vi "Swerve Drive t.vi"() -> ()   [LabVIEW 2017]
uses:
  Public/Documents/Cross The Road Electronics/Phoenix-LabVIEW/Motor Controller/Controls/CTRE_Phoenix_MotorControl_ControlMode.ctl
  <vilib>/Rock Robotics/WPI/ThirdParty/Phoenix-LabVIEW/Pigeon IMU/CTRE_PigeonIMU_TareType.ctl
  <extravilib>/ChannelInstances/Tag-dbl/Read With Abort.vi
  <extravilib>/ChannelInstances/Tag-a[.](dbl)/Read With Abort.vi
  <extravilib>/ChannelInstances/Tag-a[.](dbl)/Write With Abort.vi
  <extravilib>/ChannelInstances/Tag-dbl/Write With Abort.vi
  <extravilib>/ChannelInstances/Tag-dbl/Instantiate.vi
  <vilib>/Rock Robotics/Network Tables/NT Read Number.vi
  Robot Global Data.vi
  <extravilib>/ChannelInstances/Tag-dbl/Endpoint.vi
  <vilib>/Rock Robotics/WPI/ThirdParty/Phoenix-LabVIEW/Pigeon IMU/CTRE_PigeonIMU_GetYPR.vi
  <vilib>/Rock Robotics/Network Tables/NT Write Number.vi
  <extravilib>/ChannelInstances/Tag-a[.](dbl)/Instantiate.vi
  <extravilib>/ChannelInstances/Tag-dbl/EndpointRead.vi
  <vilib>/Rock Robotics/WPI/ThirdParty/Phoenix-LabVIEW/Motor Controller/Get/CTRE_Phoenix_MotorController_GetSelectedSensorData.vi
  <extravilib>/ChannelInstances/Tag-a[.](dbl)/Endpoint.vi
  <vilib>/Rock Robotics/Network Tables/NT Write Numeric Array.vi
  <extravilib>/ChannelInstances/Tag-a[.](dbl)/EndpointRead.vi
  <vilib>/addons/control/pid/pid.llb/PID (DBL).vi
  <extravilib>/ChannelInstances/Tag-dbl.lvlib
  <extravilib>/ChannelInstances/Tag-a[.](dbl).lvlib
  <vilib>/ptbypt/NI_PtbyPt.lvlib
  <vilib>/addons/control/pid/NI_PID_pid.lvlib
panel:
  in  "Limelight PID gains":T1={"proportional gain (Kc)"=0.035, "integral time (Ti, min)"=0.0, "derivative time (Td, min)"=0.0}
  out "Loop 3":u32=30
  out "Loop 2":u32=30
  out "Loop 1":u32=20
  in  "Rot. Point X":dbl
  in  "Rot. Point Y":dbl
  in  "Robot Width":dbl=21.125
  in  "Robot Length":dbl=22.0
  # "SWERVE DRIVE\nVersion 6.2\nCory Lynch\nChris Garuti\nGavin Popkin\nKaitlyn Sandor\nApple Pi Robotics\nTeam 2067"
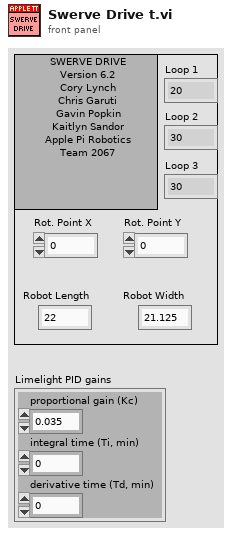
[diagram p1: front panel]
types:
  T1 = cluster{"proportional gain (Kc)":dbl, "integral time (Ti, min)":dbl, "derivative time (Td, min)":dbl}
  T2 = typedef "CTRE_PigeonIMU_DeviceRef.ctl" = cluster{"DeviceStatus":errorcluster, "Device Number":u8, "Type":T3, "Device ID":u32, "Handle":u64, "UsageFrame":u32, "Library Path":path}
  T3 = typedef "CTRE_PigeonIMU_ConnectionType.ctl" = u32
  T4 = typedef "CTRE_PigeonIMU_TareType.ctl" = u8
  T5 = typedef "Tag-dbl.lvlib/))Channel.ctl" = refnum<queue>
  T6 = typedef "WPI_MotorControlDeviceRef.ctl" = cluster{"DeviceStatus":errorcluster, "Type":T7, "PWM":cluster{"PWM Channel":T8, "DeadBand":T9}, "CAN":cluster{"Device Number":u8, "SetOutput VI Ref":variant, "GetOutput VI Ref":variant, "Enable VI Ref":variant, "Disable VI Ref":variant, "Data":variant}, "Invert":bool, "DIO PWM":cluster{"PWM \"Enable\" Channel":T8, "DIOChannel":T10, "PWM Rate":dbl}}
  T7 = typedef "WPI_MotorControlType.ctl" = enum16{"PWM", "CAN", "DIO PWM"}
  T8 = typedef "FPGA_DIOPWMChannel.ctl" = enum8{"PWM 0", "PWM 1", "PWM 2", "PWM 3", "PWM 4", "PWM 5", "PWM 6", "PWM 7", "PWM 8", "PWM 9", "PWM MXP 0", "PWM MXP 1", "PWM MXP 2", "PWM MXP 3", "PWM MXP 4", "PWM MXP 5", "PWM MXP 6", "PWM MXP 7", "PWM MXP 8", "PWM MXP 9", "Invalid"}
  T9 = typedef "WPI_PWMDeadband.ctl" = cluster{"Name":string, "maxPositivePwm":i32, "minPositivePwm":i32, "centerPwm":i32, "maxNegativePwm":i32, "minNegativePwm":i32, "angularRange":u16}
  T10 = typedef "FPGA_DIOChannel.ctl" = enum8{"DIO 0", "DIO 1", "DIO 2", "DIO 3", "DIO 4", "DIO 5", "DIO 6", "DIO 7", "DIO 8", "DIO 9", "DIO MXP 0", "DIO MXP 1", "DIO MXP 2", "DIO MXP 3", "DIO MXP 4", "DIO MXP 5", "DIO MXP 6", "DIO MXP 7", "DIO MXP 8", "DIO MXP 9", "DIO MXP 10", "DIO MXP 11", "DIO MXP 12", "DIO MXP 13", "DIO MXP 14", "DIO MXP 15", "SPI Port CS1", "SPI Port CS2", "SPI Port CS3", "SPI Port MISO", "SPI Port MOSI", "Invalid"}
  T11 = typedef "Tag-a[.](dbl).lvlib/))Channel.ctl" = refnum<queue>
  T12 = typedef "CTRE_Phoenix_MotorControl_ControlMode.ctl" = u16
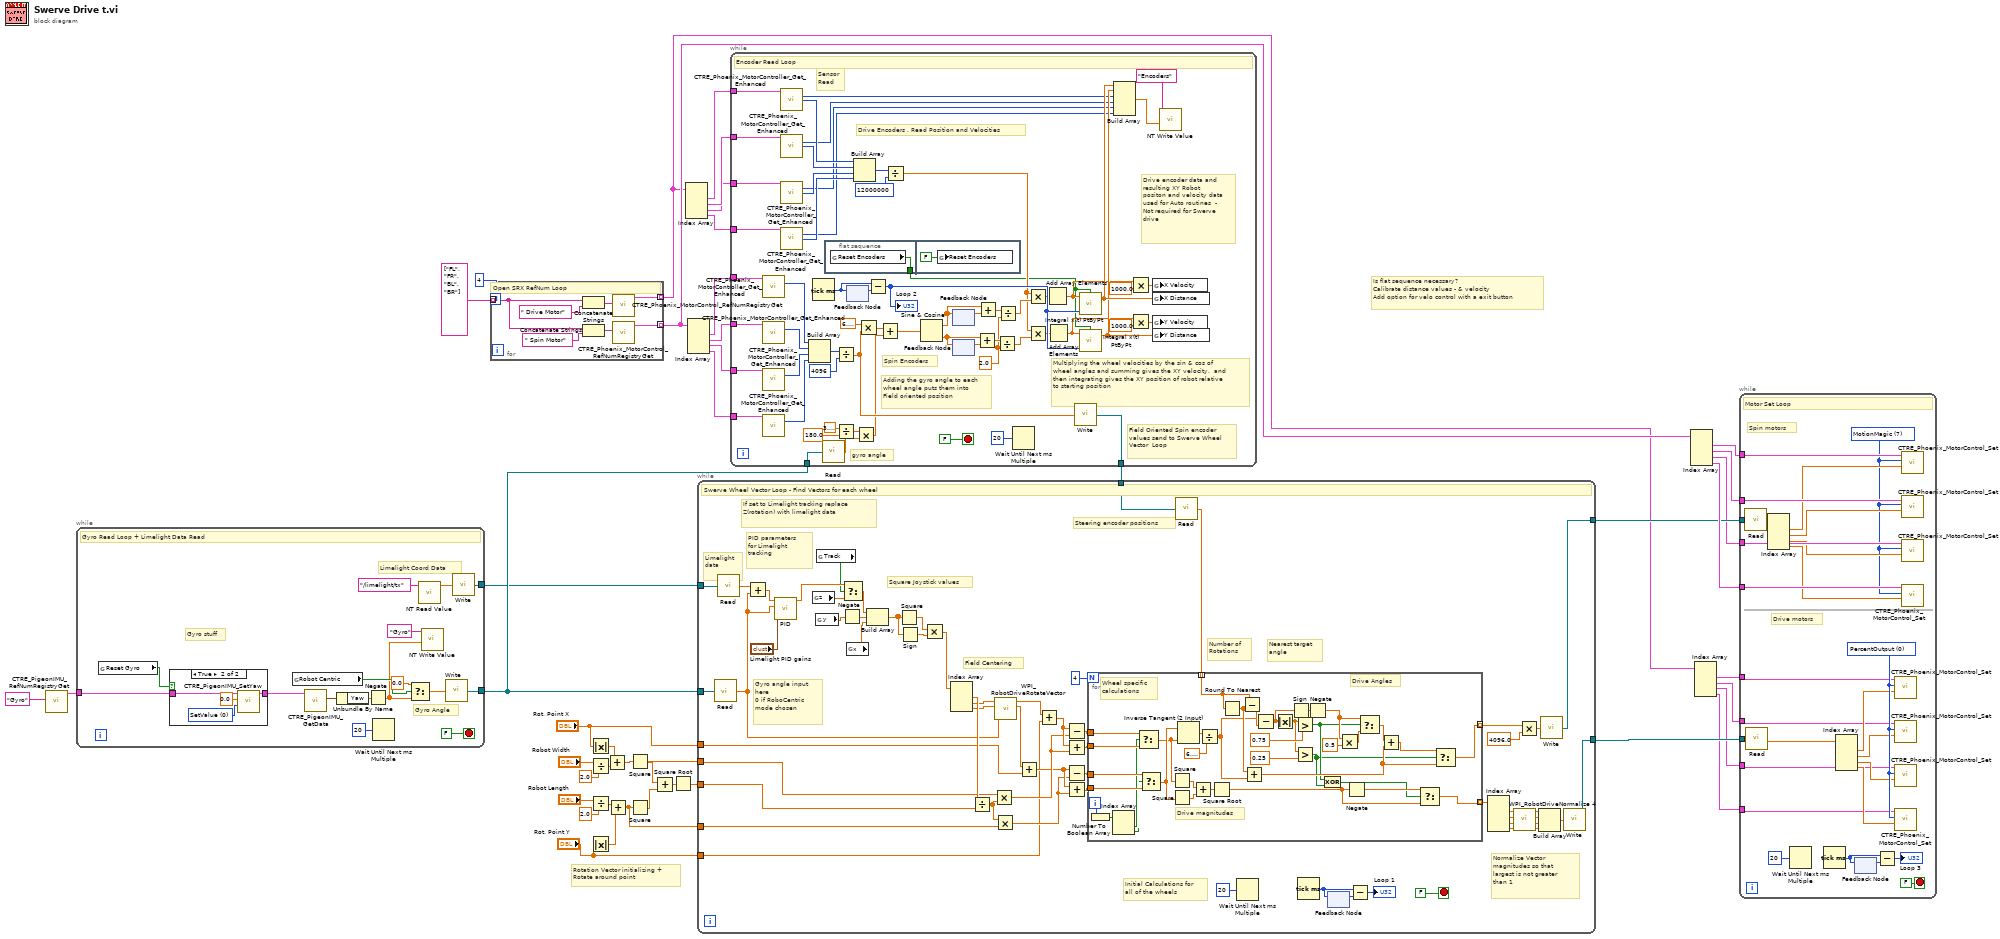
[diagram p0: block diagram]
diagram:
  # "Is flat sequence necessary?\nCalibrate distance values - & velocity\nAdd option for velo control with a exit button"
  # "Rotation Vector initializing +\nRotate around point"
  n1 = call <vilib>:"CTRE_PigeonIMU_RefNumRegistryGet.vi"("refnum name"="Gyro") -> ("PigeonIMUDevRef"=w26:T2)  [unwired: 9 in, 1 out]
  n2 = while {
    tunnel: [w57] -> w2
    tunnel: w26 -> [w51]
    tunnel: [w44] -> w1
    stop <- FALSE stop-if-true
    # "Limelight Coord Data"
    # "Gyro Angle"
    # "Gyro stuff"
    # "Gyro Read Loop + Limelight Data Read"
    n3 = global read "Robot Global Data.vi" "Reset Gyro"() -> (w47:bool)
    n4 = case shown="True" w47 {
      tunnel: w51 -> [w60 w64]
      tunnel: [w60 w63] -> w50
      frame False {
      }
      frame True {
        w62 = T4 0 items=["SetValue"=0, "AddOffset"=1, "MatchCompass"=2, "SetOffset"=255] ("TareType (SetValue)")
        n5 = call <vilib>:"CTRE_PigeonIMU_SetYaw.vi"("TareType (SetValue)"=w62, "Value"=0.0, "PigeonIMUDevRef"=w64) -> ("PigeonIMUDevRef"=w63:T2)  [unwired: 7 in, 1 out]
      }
    }
    n6 = global read "Robot Global Data.vi" "Robot Centric"() -> (w52:bool)
    n7 = call-poly <vilib>:"CTRE_PigeonIMU_GetData.vi"("PigeonIMUDevRef"=w50) -> ("Yaw Pitch Roll"=w54:cluster{"Yaw":dbl, "Pitch":dbl, "Roll":dbl})  [unwired: 8 in, 2 out]
    n8 = Unbundle By Name(w54) -> ("Yaw"=w53:dbl)
    n9 = Negate(x=w53) -> (-x=w48:dbl)
    n10 = Wait Until Next ms Multiple(millisecond multiple=u32 20) -> ()  [unwired: 1 out]
    n11 = Select(t=0.0, s=w52, f=w48) -> (s? t:f=w58:dbl)
    n12 = call-poly <vilib>:"NT Read Value.vi"("Name"="/limelight/tx") -> ("Numeric"=w45:dbl)  [unwired: 9 in, 1 out]
    n13 = call-poly <vilib>:"NT Write Value.vi"("Numeric"=w48, "Name"="Gyro") -> ()  [unwired: 9 in, 1 out]
    n14 = call <extravilib>:"Write.vi"("element"=w58) -> ("channel"=w57:T5)  [unwired: 1 out]
    n15 = call <extravilib>:"Write.vi"("element"=w45) -> ("channel"=w44:T5)  [unwired: 1 out]
  }
  n16 = for {
    N: 4 -> [_]
    tunnel: string[] ["FL", "FR", "BL", "BR"] -> [w71] mode=indexing
    tunnel: [w65] -> w7 mode=indexing
    tunnel: [w66] -> w36 mode=indexing
    # "Open SRX RefNum Loop"
    n17 = Concatenate Strings(w71, " Drive Motor") -> (w69:string)
    n18 = Concatenate Strings(w71, " Spin Motor" ("refnum name")) -> (w70:string)
    n19 = call <vilib>:"CTRE_Phoenix_MotorControl_RefNumRegistryGet.vi"("refnum name"=w69) -> ("PhoenixMotorControlDevRef"=w65:T6)  [unwired: 9 in, 1 out]
    n20 = call <vilib>:"CTRE_Phoenix_MotorControl_RefNumRegistryGet.vi"("refnum name"=w70) -> ("PhoenixMotorControlDevRef"=w66:T6)  [unwired: 9 in, 1 out]
  }
  n21 = Absolute Value(x="Rot. Point X") -> (abs(x)=w11:dbl)
  n22 = Divide(x="Robot Width", y=2.0) -> (x/y=w22:dbl)
  n23 = Divide(x="Robot Length", y=2.0) -> (x/y=w23:dbl)
  n24 = Absolute Value(x="Rot. Point Y") -> (abs(x)=w24:dbl)
  n25 = Add(x=w11, y=w22) -> (x+y=w14:dbl)
  n26 = Add(x=w23, y=w24) -> (x+y=w10:dbl)
  n27 = Square(x=w14) -> (x^2=w19:dbl)
  n28 = Square(x=w10) -> (x^2=w20:dbl)
  n29 = Add(x=w19, y=w20) -> (x+y=w18:dbl)
  n30 = Square Root(x=w18) -> (sqrt(x)=w12:dbl)
  n31 = Index Array(array=w7) -> (element #1=w6:T6, element #2=w5:T6, element #3=w4:T6, element #4=w3:T6)  [unwired: 4 in]
  n32 = Index Array(array=w36) -> (element #1=w40:T6, element #2=w39:T6, element #3=w38:T6, element #4=w37:T6)  [unwired: 4 in]
  n33 = while {
    tunnel: w40 -> [w133]
    tunnel: w39 -> [w130]
    tunnel: w38 -> [w126]
    tunnel: w37 -> [w125]
    tunnel: [w120] -> w8
    tunnel: w6 -> [w119]
    tunnel: w5 -> [w118]
    tunnel: w4 -> [w117]
    tunnel: w3 -> [w116]
    tunnel: w2 -> [w109]
    stop <- FALSE stop-if-true
    w87 = 2.0
    # "Drive encoder data and resulting XY Robot positon and velocity data used for Auto routines  - Not required for Swerve drive"
    # "Field Oriented Spin encoder values send to Swerve Wheel Vector  Loop"
    # "Spin Encoders"
    # "Drive Encoders , Read Position and Velocities"
    # "gyro angle"
    # "Multiplying the wheel velocities by the sin & cos of wheel angles and summing gives the XY velocity,  and then integrating gives the XY position of robot relative to starting position"
    # "Adding the gyro angle to each wheel angle puts them into Field oriented position"
    # "Sensor\nRead"
    # "Encoder Read Loop"
    n34 = call-poly <vilib>:"CTRE_Phoenix_MotorController_Get_Enhanced.vi"("PhoenixMotorControlDevRef"=w133) -> ("Position (Raw Sensor Units)"=w131:i32)  [unwired: 11 in, 3 out]
    n35 = call-poly <vilib>:"CTRE_Phoenix_MotorController_Get_Enhanced.vi"("PhoenixMotorControlDevRef"=w130) -> ("Position (Raw Sensor Units)"=w129:i32)  [unwired: 11 in, 3 out]
    n36 = call-poly <vilib>:"CTRE_Phoenix_MotorController_Get_Enhanced.vi"("PhoenixMotorControlDevRef"=w126) -> ("Position (Raw Sensor Units)"=w127:i32)  [unwired: 11 in, 3 out]
    n37 = call-poly <vilib>:"CTRE_Phoenix_MotorController_Get_Enhanced.vi"("PhoenixMotorControlDevRef"=w125) -> ("Position (Raw Sensor Units)"=w128:i32)  [unwired: 11 in, 3 out]
    n38 = call-poly <vilib>:"CTRE_Phoenix_MotorController_Get_Enhanced.vi"("PhoenixMotorControlDevRef"=w119) -> ("Position (Raw Sensor Units)"=w77:i32, "Velocity (Raw Sensor Units per 100 ms)"=w80:i32)  [unwired: 11 in, 2 out]
    n39 = call-poly <vilib>:"CTRE_Phoenix_MotorController_Get_Enhanced.vi"("PhoenixMotorControlDevRef"=w118) -> ("Position (Raw Sensor Units)"=w76:i32, "Velocity (Raw Sensor Units per 100 ms)"=w81:i32)  [unwired: 11 in, 2 out]
    n40 = call-poly <vilib>:"CTRE_Phoenix_MotorController_Get_Enhanced.vi"("PhoenixMotorControlDevRef"=w117) -> ("Position (Raw Sensor Units)"=w75:i32, "Velocity (Raw Sensor Units per 100 ms)"=w82:i32)  [unwired: 11 in, 2 out]
    n41 = call-poly <vilib>:"CTRE_Phoenix_MotorController_Get_Enhanced.vi"("PhoenixMotorControlDevRef"=w116) -> ("Position (Raw Sensor Units)"=w74:i32, "Velocity (Raw Sensor Units per 100 ms)"=w83:i32)  [unwired: 11 in, 2 out]
    n42 = Build Array(w131, w129, w127, w128) -> (w121:i32[])
    n43 = Tick Count (ms)() -> (millisecond timer value=w124:u32)
    n44 = call <extravilib>:"Read.vi"("channel"=w109) -> ("element"=w106:dbl)  [unwired: 1 in, 1 out]
    n45 = flat-sequence {
      tunnel: [w135] -> w72
      frame #0 {
        n46 = global read "Robot Global Data.vi" "Reset Encoders"() -> (w135:bool)
      }
      frame #1 {
        n47 = global write "Robot Global Data.vi" "Reset Encoders"(FALSE ("Reset Encoders")) -> ()
      }
    }
    n48 = Divide(x=w121, y=4096) -> (x/y=w115:dbl[])
    n49 = Divide(x=3.141592653589793, y=180.0) -> (x/y=w108:dbl)
    n50 = feedback #1() -> (w123:u32)  [unwired: 1 in]
    n51 = feedback-in #1(w124) -> ()
    n52 = Build Array(w80, w81, w82, w83) -> (w84:i32[])
    n53 = Multiply(x=w108, y=w106) -> (x*y=w107:dbl)
    n54 = Multiply(x=6.283185307179586, y=w115) -> (x*y=w112:dbl[])
    n55 = Subtract(x=w124, y=w123) -> (x-y=w103:u32)
    "Loop 2" <- w103
    n56 = Add(x=w112, y=w107) -> (x+y=w113:dbl[])
    n57 = Divide(x=w84, y=12000000) -> (x/y=w73:dbl[])
    n58 = Sine & Cosine(0:w113) -> (1:w93:dbl[], 2:w88:dbl[])
    n59 = feedback #2() -> (w94:dbl[])  [unwired: 1 in]
    n60 = feedback-in #2(w93) -> ()
    n61 = feedback #3() -> (w89:dbl[])  [unwired: 1 in]
    n62 = feedback-in #3(w88) -> ()
    n63 = Add(x=w88, y=w89) -> (x+y=w90:dbl[])
    n64 = Add(x=w93, y=w94) -> (x+y=w91:dbl[])
    n65 = Divide(x=w90, y=w87) -> (x/y=w86:dbl[])
    n66 = Divide(x=w91, y=w87) -> (x/y=w92:dbl[])
    n67 = Wait Until Next ms Multiple(millisecond multiple=u32 20) -> ()  [unwired: 1 out]
    n68 = Multiply(x=w73, y=w92) -> (x*y=w102:dbl[])
    n69 = Multiply(x=w73, y=w86) -> (x*y=w101:dbl[])
    n70 = Add Array Elements(numeric array=w102) -> (sum=w98:dbl)
    n71 = Add Array Elements(numeric array=w101) -> (sum=w97:dbl)
    n72 = call <extravilib>:"Write.vi"("element"=w115) -> ("channel"=w120:T11)  [unwired: 1 out]
    n73 = call <vilib>:"Integral x(t) PtByPt.vi"("initialize"=w72, "dt"=w103, "x"=w98) -> ("integral x(t)"=w105:dbl)  [unwired: 1 in, 1 out]
    n74 = call <vilib>:"Integral x(t) PtByPt.vi"("initialize"=w72, "dt"=w103, "x"=w97) -> ("integral x(t)"=w104:dbl)  [unwired: 1 in, 1 out]
    n75 = Build Array(w105, w104, w77, w76, w75, w74) -> (w79:dbl[])
    n76 = Multiply(x=w98, y=1000.0) -> (x*y=w96:dbl)
    n77 = Multiply(x=w97, y=1000.0) -> (x*y=w95:dbl)
    n78 = global write "Robot Global Data.vi" "X Velocity"(w96) -> ()
    n79 = global write "Robot Global Data.vi" "X Distance"(w105) -> ()
    n80 = global write "Robot Global Data.vi" "Y Velocity"(w95) -> ()
    n81 = global write "Robot Global Data.vi" "Y Distance"(w104) -> ()
    n82 = call-poly <vilib>:"NT Write Value.vi"("Numeric Array"=w79, "Name"="Encoders") -> ()  [unwired: 9 in, 1 out]
  }
  n83 = while {
    tunnel: w2 -> [w171]
    tunnel: w8 -> [w170]
    tunnel: [w167] -> w43
    tunnel: [w165] -> w28
    tunnel: w14 -> [w154]
    tunnel: "Rot. Point X" -> [w153]
    tunnel: w10 -> [w152]
    tunnel: w12 -> [w151]
    tunnel: "Rot. Point Y" -> [w150]
    tunnel: w1 -> [w148]
    stop <- FALSE stop-if-true
    # "Limelight data"
    # "Steering encoder positions"
    # "PID parameters for Limelight tracking"
    # "Square Joystick values"
    # "Normalize Vector magnitudes so that largest is not greater than 1"
    # "If set to Limelight tracking replace Z(rotation) with limelight data"
    # "Gyro angle input here\n0 if RoboCentric mode chosen"
    # "Field Centering"
    # "Number of\nRotations"
    # "Nearest target\nangle"
    # "Initial Calculations for\nall of the wheels"
    # "Swerve Wheel Vector Loop - Find Vectors for each wheel"
    n84 = call <extravilib>:"Read.vi"("channel"=w171) -> ("element"=w137:dbl)  [unwired: 1 in, 1 out]
    n85 = call <extravilib>:"Read.vi"("channel"=w148) -> ("element"=w147:dbl)  [unwired: 1 in, 1 out]
    n86 = Add(x=w147, y=w137) -> (x+y=w146:dbl)
    n87 = call-poly <vilib>:"PID.vi"("PID gains"="Limelight PID gains", "process variable"=w137, "setpoint"=w146) -> ("output"=w143:dbl)  [unwired: 7 in, 1 out]
    n88 = global read "Robot Global Data.vi" "z"() -> (w164:dbl)
    n89 = global read "Robot Global Data.vi" "y"() -> (w163:dbl)
    n90 = global read "Robot Global Data.vi" "Track"() -> (w142:bool)
    n91 = Negate(x=w163) -> (-x=w138:dbl)
    n92 = Select(t=w143, s=w142, f=w164) -> (s? t:f=w144:dbl)
    n93 = global read "Robot Global Data.vi" "x"() -> (w162:dbl)
    n94 = Build Array(w144, w138, w162) -> (w141:dbl[])
    n95 = Square(x=w141) -> (x^2=w139:dbl[])
    n96 = Sign(1:w141) -> (0:w140:dbl[])
    n97 = Multiply(x=w139, y=w140) -> (x*y=w161:dbl[])
    n98 = Index Array(array=w161) -> (element #1=w184:dbl, element #2=w183:dbl, element #3=w182:dbl)  [unwired: 3 in]
    n99 = Divide(x=w184, y=w151) -> (x/y=w195:dbl)
    n100 = Multiply(x=w154, y=w195) -> (x*y=w192:dbl)
    n101 = Multiply(x=w195, y=w152) -> (x*y=w188:dbl)
    n102 = call <vilib>:"WPI_RobotDriveRotateVector.vi"("Angle"=w137, "X"=w182, "Y"=w183) -> ("X'"=w187:dbl, "Y'"=w194:dbl)  [unwired: 7 out]
    n103 = Add(x=w187, y=w153) -> (x+y=w189:dbl)
    n104 = Add(x=w194, y=w150) -> (x+y=w193:dbl)
    n105 = Subtract(x=w193, y=w192) -> (x-y=w191:dbl)
    n106 = Add(x=w193, y=w192) -> (x+y=w190:dbl)
    n107 = Subtract(x=w189, y=w188) -> (x-y=w186:dbl)
    n108 = Add(x=w189, y=w188) -> (x+y=w185:dbl)
    n109 = call <extravilib>:"Read.vi"("channel"=w170) -> ("element"=w149:dbl[])  [unwired: 1 in, 1 out]
    n110 = for {
      N: 4 -> [_]
      tunnel: [w196] -> w181 mode=indexing
      tunnel: w191 -> [w221]
      tunnel: w190 -> [w222]
      tunnel: w186 -> [w224]
      tunnel: w185 -> [w223]
      tunnel: [w199] -> w160 mode=indexing
      tunnel: w149 -> [w198] mode=indexing
      i -> [w226]
      # "Drive Angles"
      # "Drive magnitudes"
      # "Wheel specific\ncalculations"
      n111 = Number To Boolean Array(number=w226) -> (Boolean array=w225:bool[])
      n112 = Index Array(array=w225) -> (element #1=w220:bool, element #2=w219:bool)  [unwired: 2 in]
      n113 = Select(t=w221, s=w220, f=w222) -> (s? t:f=w217:dbl)
      n114 = Select(t=w224, s=w219, f=w223) -> (s? t:f=w218:dbl)
      n115 = Square(x=w217) -> (x^2=w231:dbl)
      n116 = Square(x=w218) -> (x^2=w232:dbl)
      n117 = Inverse Tangent (2 Input)(1:w217, 2:w218) -> (0:w227:dbl)
      n118 = Add(x=w231, y=w232) -> (x+y=w230:dbl)
      n119 = Divide(x=w227, y=6.283185307179586) -> (x/y=w210:dbl)
      n120 = Square Root(x=w230) -> (sqrt(x)=w229:dbl)
      n121 = Round To Nearest(number=w198) -> (nearest integer value=w211:dbl)
      n122 = Subtract(x=w198, y=w211) -> (x-y=w216:dbl)
      n123 = Add(x=w211, y=w210) -> (x+y=w206:dbl)
      n124 = Subtract(x=w210, y=w216) -> (x-y=w212:dbl)
      n125 = Absolute Value(x=w212) -> (abs(x)=w214:dbl)
      n126 = Sign(1:w212) -> (0:w208:dbl)
      n127 = Greater?(x=w214, y=0.75) -> (0:w204:bool)
      n128 = Greater?(x=w214, y=0.25) -> (0:w203:bool)
      n129 = Negate(x=w208) -> (-x=w205:dbl)
      n130 = Exclusive Or(1:w203, 2:w204) -> (0:w197:bool)
      n131 = Multiply(x=w205, y=0.5) -> (x*y=w202:dbl)
      n132 = Negate(x=w229) -> (-x=w200:dbl)
      n133 = Select(t=w205, s=w204, f=w202) -> (s? t:f=w207:dbl)
      n134 = Add(x=w207, y=w206) -> (x+y=w201:dbl)
      n135 = Select(t=w200, s=w197, f=w229) -> (s? t:f=w196:dbl)
      n136 = Select(t=w201, s=w203, f=w206) -> (s? t:f=w199:dbl)
    }
    n137 = Wait Until Next ms Multiple(millisecond multiple=u32 20) -> ()  [unwired: 1 out]
    n138 = Tick Count (ms)() -> (millisecond timer value=w156:u32)
    n139 = feedback-in #4(w156) -> ()
    n140 = feedback #4() -> (w157:u32)  [unwired: 1 in]
    n141 = Subtract(x=w156, y=w157) -> (x-y=→"Loop 1":u32)
    n142 = Index Array(array=w181) -> (element #1=w180:dbl, element #2=w179:dbl, element #3=w178:dbl, element #4=w177:dbl)  [unwired: 4 in]
    n143 = call <vilib>:"WPI_RobotDriveNormalize 4.vi"("D"=w177, "C"=w178, "B"=w179, "A"=w180) -> ("D'"=w172:dbl, "C'"=w173:dbl, "B'"=w174:dbl, "A'"=w175:dbl)
    n144 = Multiply(x=w160, y=4096.0) -> (x*y=w159:dbl[])
    n145 = Build Array(w175, w174, w173, w172) -> (w168:dbl[])
    n146 = call <extravilib>:"Write.vi"("element"=w159) -> ("channel"=w165:T11)  [unwired: 1 out]
    n147 = call <extravilib>:"Write.vi"("element"=w168) -> ("channel"=w167:T11)  [unwired: 1 out]
  }
  n148 = Index Array(array=w36) -> (element #1=w35:T6, element #2=w34:T6, element #3=w27:T6, element #4=w33:T6)  [unwired: 4 in]
  n149 = Index Array(array=w7) -> (element #1=w32:T6, element #2=w31:T6, element #3=w30:T6, element #4=w29:T6)  [unwired: 4 in]
  n150 = while {
    tunnel: w43 -> [w257]
    tunnel: w35 -> [w251]
    tunnel: w32 -> [w247]
    tunnel: w34 -> [w250]
    tunnel: w27 -> [w249]
    tunnel: w33 -> [w248]
    tunnel: w31 -> [w246]
    tunnel: w30 -> [w245]
    tunnel: w29 -> [w244]
    tunnel: w28 -> [w242]
    stop <- FALSE stop-if-true
    w233 = T12 7 items=["PercentOutput"=0, "Position"=1, "Velocity"=2, "Current"=3, "Follower"=5, "MotionProfile"=6, "MotionMagic"=7, "MotionMagicArc"=8, "MotionProfileArc"=10, "Disabled"=15] ("Control Mode")
    w258 = T12 0 items=["PercentOutput"=0, "Position"=1, "Velocity"=2, "Current"=3, "Follower"=5, "MotionProfile"=6, "MotionMagic"=7, "MotionMagicArc"=8, "MotionProfileArc"=10, "Disabled"=15] ("Control Mode")
    # "Drive motors"
    # "Spin motors"
    # "Motor Set Loop"
    n151 = call <extravilib>:"Read.vi"("channel"=w242) -> ("element"=w241:dbl[])  [unwired: 1 in, 1 out]
    n152 = call <extravilib>:"Read.vi"("channel"=w257) -> ("element"=w256:dbl[])  [unwired: 1 in, 1 out]
    n153 = Index Array(array=w241) -> (element #1=w240:dbl, element #2=w237:dbl, element #3=w238:dbl, element #4=w239:dbl)  [unwired: 4 in]
    n154 = Wait Until Next ms Multiple(millisecond multiple=u32 20) -> ()  [unwired: 1 out]
    n155 = Tick Count (ms)() -> (millisecond timer value=w235:u32)
    n156 = Index Array(array=w256) -> (element #1=w255:dbl, element #2=w254:dbl, element #3=w253:dbl, element #4=w252:dbl)  [unwired: 4 in]
    n157 = feedback #5() -> (w234:u32)  [unwired: 1 in]
    n158 = feedback-in #5(w235) -> ()
    n159 = Subtract(x=w235, y=w234) -> (x-y=→"Loop 3":u32)
    n160 = call <vilib>:"CTRE_Phoenix_MotorControl_Set.vi"("Output"=w255, "Control Mode"=w258, "PhoenixMotorControlDevRef"=w247) -> ()  [unwired: 7 in, 2 out]
    n161 = call <vilib>:"CTRE_Phoenix_MotorControl_Set.vi"("Output"=w254, "Control Mode"=w258, "PhoenixMotorControlDevRef"=w246) -> ()  [unwired: 7 in, 2 out]
    n162 = call <vilib>:"CTRE_Phoenix_MotorControl_Set.vi"("Output"=w253, "Control Mode"=w258, "PhoenixMotorControlDevRef"=w245) -> ()  [unwired: 7 in, 2 out]
    n163 = call <vilib>:"CTRE_Phoenix_MotorControl_Set.vi"("Output"=w252, "Control Mode"=w258, "PhoenixMotorControlDevRef"=w244) -> ()  [unwired: 7 in, 2 out]
    n164 = call <vilib>:"CTRE_Phoenix_MotorControl_Set.vi"("Output"=w240, "Control Mode"=w233, "PhoenixMotorControlDevRef"=w251) -> ()  [unwired: 7 in, 2 out]
    n165 = call <vilib>:"CTRE_Phoenix_MotorControl_Set.vi"("Output"=w237, "Control Mode"=w233, "PhoenixMotorControlDevRef"=w250) -> ()  [unwired: 7 in, 2 out]
    n166 = call <vilib>:"CTRE_Phoenix_MotorControl_Set.vi"("Output"=w238, "Control Mode"=w233, "PhoenixMotorControlDevRef"=w249) -> ()  [unwired: 7 in, 2 out]
    n167 = call <vilib>:"CTRE_Phoenix_MotorControl_Set.vi"("Output"=w239, "Control Mode"=w233, "PhoenixMotorControlDevRef"=w248) -> ()  [unwired: 7 in, 2 out]
  }
